vi "SendString.vi"(8 "error in (no error)":errorcluster, 10 "Message":string, 11 "TCP_Server_Connection_Handler in":refnum<class "TCP_Server_Connection_Handler.lvclass">) -> (0 "error out":errorcluster, 3 "TCP_Server_Connection_Handler out":refnum<class "TCP_Server_Connection_Handler.lvclass">)   [LabVIEW 2023, in "TCP_Server_Connection_Handler.lvlib" / "TCP_Server_Connection_Handler.lvclass"]
uses:
  TCP_Server_Connection_Handler.lvclass
  TCP_Server_Connection_Handler.lvclass/TCP_Server_Connection_Handler.ctl
  <vilib>/ActorFramework/Actor/Actor.lvclass/Actor.ctl
  <vilib>/ActorFramework/Message Enqueuer/Message Enqueuer.lvclass/Message Enqueuer.ctl
  <vilib>/ActorFramework/Message Enqueuer/Init from Existing Queue.vi
  <vilib>/ActorFramework/Message Enqueuer/Enqueue.vi
  <vilib>/ActorFramework/Stop Msg/Stop Msg.lvclass
  <vilib>/ActorFramework/Message Priority Queue/Priority Enqueue.vi
  <vilib>/ActorFramework/Message Enqueuer/Message Enqueuer.lvclass
  <vilib>/ActorFramework/Actor/Actor.lvclass
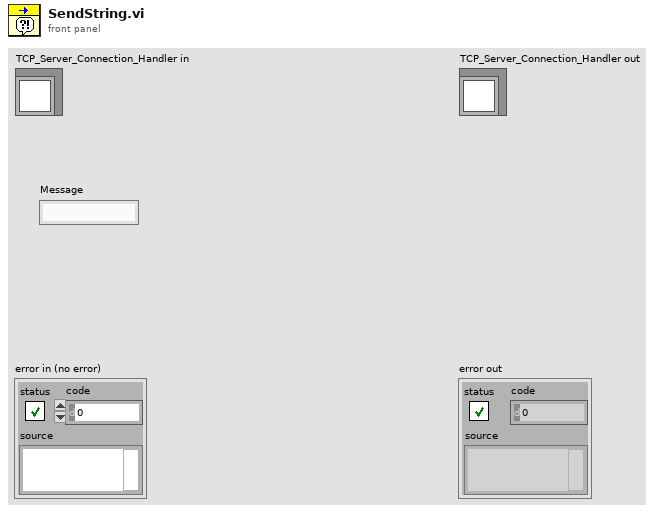
[diagram p1: front panel]
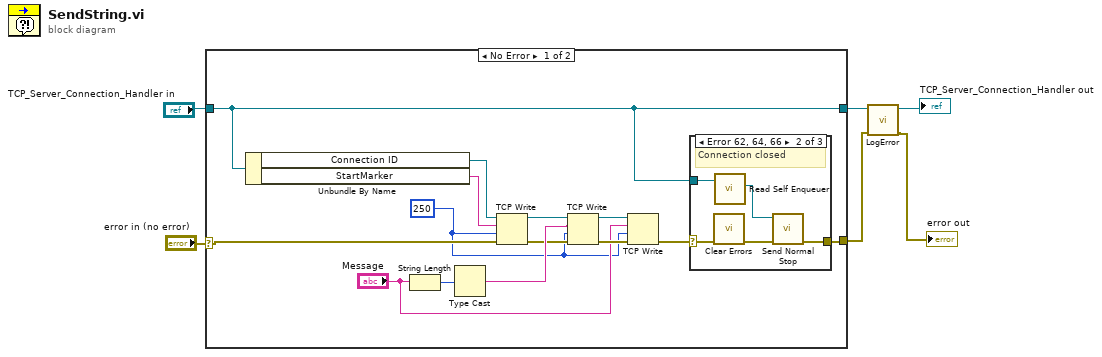
[diagram p0: block diagram]
diagram:
  n1 = case shown="No Error" "error in (no error)" {
    selector: "error in (no error)" -> [w11 w29]
    tunnel: [w8 w29] -> w2
    tunnel: [w9 w28] -> w4
    tunnel: "TCP_Server_Connection_Handler in" -> [w9 w28]
    frame No Error {
      w7 = 250 ("timeout ms (25000)")
      n2 = Unbundle By Name(w9) -> ("Connection ID"=w12:refnum<k5>, "StartMarker"=w14:string)
      n3 = String Length(string="Message") -> (length=w20:i32)
      n4 = Type Cast(x=w20) -> (*(type *) &x=w19:string)  [unwired: 1 in]
      n5 = TCP Write(connection ID=w12, data in=w14, error in (no error)=w11, 9:w7) -> (connection ID out=w15:refnum<k5>, error out=w13:errorcluster)  [unwired: 1 out]
      n6 = TCP Write(connection ID=w15, data in=w19, error in (no error)=w13, 9:w7) -> (connection ID out=w18:refnum<k5>, error out=w17:errorcluster)  [unwired: 1 out]
      n7 = TCP Write(connection ID=w18, data in="Message", error in (no error)=w17, 9:w7) -> (error out=w10:errorcluster)  [unwired: 2 out]
      n8 = case shown="Error 62, 64, 66" w10 {
        selector: w10 -> [w21 w24 w27]
        tunnel: w9 -> [_ w26 _]
        tunnel: [w21 w22 w27] -> w8
        frame No Error {
        }
        frame Error {
          # "Connection closed"
          n9 = call <vilib>:"Clear Errors.vi"("error in (no error)"=w24) -> ("error out"=w23:errorcluster)  [unwired: 5 in, 1 out]
          n10 = call <vilib>:"Read Self Enqueuer.vi"("Actor"=w26) -> ("Self Enqueuer"=w25:refnum<class "Message Enqueuer.lvclass">)  [unwired: 10 in]
          n11 = call <vilib>:"Send Normal Stop.vi"("error in (no error)"=w23, "Message Enqueuer"=w25) -> ("error out"=w22:errorcluster)  [unwired: 9 in]
        }
        frame Default {
        }
      }
    }
    frame Error {
    }
  }
  n12 = call "LogError.vi"("error in (no error)"=w2, "TCP_Server_Connection_Handler in"=w4) -> ("error out"=→"error out":errorcluster, "TCP_Server_Connection_Handler out"=→"TCP_Server_Connection_Handler out":refnum<class "TCP_Server_Connection_Handler.lvclass">)  [unwired: 8 in]
